vi "AlliGator 2-Exp + IRF Convolution Fit v2.vi"(0 "Decay":cluster{"t Array":dbl[], "Data Array":dbl[]}, 5 "IRF":cluster{"t Array":dbl[], "IRF Array":dbl[]}, 9 "Fit Options":T9={"Show Fit Residuals"=TRUE, "Fit Model"=enum."1-Exponential", "Residual Type"=enum."Standard", "Max Decay Percentile"=0.0, "Min Decay Percentile"=0.0, "Show Full Decay"=TRUE, "Weights"=enum."Unweighted", "Fitting Method"=enum."Least Square", "Compute Parameter Uncertainties"=TRUE, "Periodic Boundaries"=TRUE, "Model Calculation"=enum."Simulation", "Period"=1.2500000000000001e-08, "Termination Criteria"={"Max Iterations"=1000, "Max Function Calls"=0, "Max Time"=1000.0, "Function Tolerance"=1e-06, "Parameter Tolerance"=1e-06, "Gradient Tolerance"=0.0, "Min Lambda"=1e-06, "Max Lambda"=1e-06, "Initial Tick Count"=0}, "Offset Resolution"=1.2500000000000001e-08, "Use Local IRF"=TRUE, "Fitting Algorithm"=enum."Levenberg-Marquardt"} {"Offset Resolution" min=0.0; "Period" min=0.0; "Min Decay Percentile" min=0.0 max=1.0; "Max Decay Percentile" min=0.0 max=100.0}, 11 "error in (no error)":errorcluster, 12 "parameter bounds":T8) -> (4 "Fitted Decay":cluster{"t Array":dbl[], "Fitted Array":dbl[]}, 6 "Residuals":cluster{"t Array":dbl[], "Residual Array":dbl[]}, 8 "Fit Output":T2={"best nonlinear fit"=[], "best fit parameters"=[], "R^2"=0.0, "RMSE"=0.0, "error out"={"status"=FALSE, "code"=0, "source"=""}, "Fitting Method"=enum."Least Square", "number of function calls"=0, "number of iterations"=0, "covariance"=[], "Chi 2"=0.0, "DOF"=0, "Fit Convergence Criterion"=enum."Continue", "Fitting Algorithm"=enum."Levenberg-Marquardt", "Weighted Fit"=FALSE, "Gradient"=0.0, "|Delta Chi 2|"=0.0, "|Delta Chi 2|/Chi 2"=0.0, "Max |Delta a| /|a|"=0.0, "Lambda"=-1.0, "RSS"=0.0, "AIC"=0.0, "BIC"=0.0, "Max number of function calls"=0, "Max number of iterations"=0, "IRF"={"X Array"=[], "Y Array"=[]}, "IRF Normalization Factor"=0.0, "Decay Normalization Factor"=0.0}, 10 "Delta Best Fit Parameters":dbl[](array[numeric]), 13 "Guess Parameters Options":T1=enum."User-provided (normalized)", 14 "Guess Parameters":dbl[](array[numeric]), 15 "error out":errorcluster)   [LabVIEW 2021, in "AlliGator Decay Analysis.lvlib" / "AlliGator Decay Fit.lvlib"]
doc: "Legacy code for 2-Exp decay fit."
uses:
  AlliGator Decay Fit.lvlib
  Fits/IRF(X)PSED/Decay Fit Options v2.ctl
  Fits/Decay Convolution/Decay Model.ctl
  Fits/Residual Type.ctl
  Fits/IRF(X)PSED/Fit Weights Type.ctl
  Fits/Non-linear Fitting Method v2.ctl
  Fits/Fit Calculation Method.ctl
  Fits/Non-linear Fitting Algorithm.ctl
  Fits/Non-linear Fit Output v3.ctl
  Fits/Nonlinear Fit Method.ctl
  <vilib>/Analysis/Matrix/Datatypes/RealMatrix.ctl
  Fits/Convergence Criteria.ctl
  Graphs/XY Graph/XY Plot Data.ctl
  AlliGator Guess Parameters Options.ctl
  AlliGator Settings List.ctl
  Fits/Decay Convolution/Fit Control Data.ctl
  AlliGator Variables List.ctl
  Fits/Decay Convolution/LM model function and gradient (2-Exp + IRF) v2.vi
  Phasor/Phasor Abort Parallel Computation.vi
  Fits/Decay Convolution/LM model function and gradient (2-Exp, Convolved, Periodic) v3.vi
  <vilib>/Utility/error.llb/Error Cluster From Error Code.vi
  Fits/Abort Fit Global.vi
  <vilib>/ErrorRing/Error Ring.xnode
  Time/Time.lvlib
  Fits/Fits.lvlib
  AlliGator Settings.lvlib
  Phasor/Phasor.lvlib
  AlliGator Globals, Variables & Constants.lvlib
  Error/Error.lvlib
  Graphs/XY Graph/XY Graph Add-Ons.lvlib
  <vilib>/Analysis/Matrix/NI_Matrix.lvlib
panel:
  out "CPU (s)":dbl
  out "XY Graph":T15(graph)
  # "Offset\nBaseline\nA1\ntau1\nA2\ntau2"
  # "Offset\nBaseline\nA1\ntau 1\nA2\ntau 2"
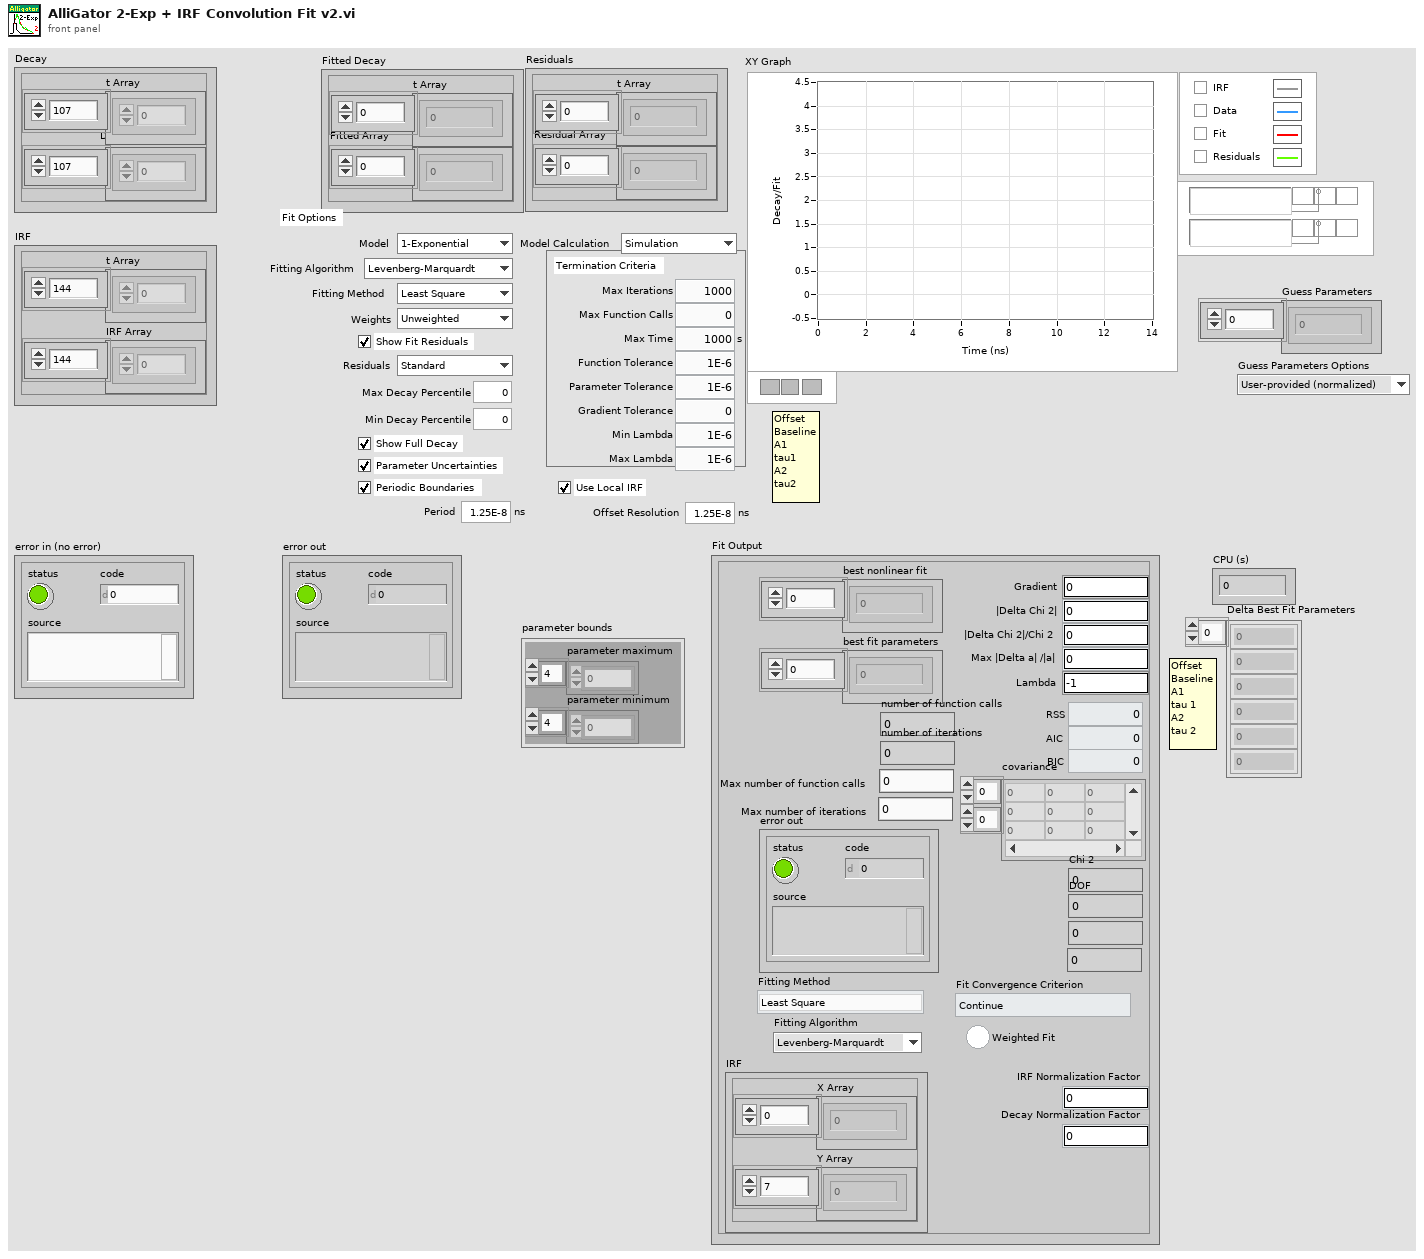
[diagram p1: front panel]
types:
  T1 = typedef "AlliGator Decay Analysis.lvlib/AlliGator Decay Fit.lvlib/AlliGator Guess Parameters Options.ctl" = enum16{"Numerically estimated", "User-provided", "User-provided (normalized)", "Last valid fitted parameters"}
  T2 = typedef "Fits.lvlib/Non-linear Fit Output v3.ctl" = cluster{"best nonlinear fit":dbl[], "best fit parameters":dbl[], "R^2":dbl, "RMSE":dbl, "error out":errorcluster, "Fitting Method":T3, "number of function calls":i32, "number of iterations":i32, "covariance":T4, "Chi 2":dbl, "DOF":i32, "Fit Convergence Criterion":T5, "Fitting Algorithm":T6, "Weighted Fit":bool, "Gradient":dbl, "|Delta Chi 2|":dbl, "|Delta Chi 2|/Chi 2":dbl, "Max |Delta a| /|a|":dbl, "Lambda":dbl, "RSS":dbl, "AIC":dbl, "BIC":dbl, "Max number of function calls":i32, "Max number of iterations":i32, "IRF":T7, "IRF Normalization Factor":dbl, "Decay Normalization Factor":dbl}
  T3 = typedef "Fits.lvlib/Nonlinear Fit Method.ctl" = enum16{"Least Square", "Least Absolute Residual", "Bisquare", "MLE"}
  T4 = typedef "NI_Matrix.lvlib/RealMatrix.ctl" = dbl[][]
  T5 = typedef "Fits.lvlib/Convergence Criteria.ctl" = enum16{"Continue", "Tolerances Exceeded", "Max Time Exceeded", "Max Iterations Exceeded", "Max Function Evaluations Exceeded", "Scale Range Exceeded"}
  T6 = typedef "Fits.lvlib/Non-linear Fitting Algorithm.ctl" = enum16{"Levenberg-Marquardt", "Trust-Region Dogleg"}
  T7 = typedef "XY Graph Add-Ons.lvlib/XY Plot Data.ctl" = cluster{"X Array":dbl[], "Y Array":dbl[]}
  T8 = cluster{"parameter minimum":dbl[], "parameter maximum":dbl[]}
  T9 = typedef "Fits.lvlib/Decay Fit Options v2.ctl" = cluster{"Show Fit Residuals":bool, "Fit Model":T10, "Residual Type":T11, "Max Decay Percentile":dbl, "Min Decay Percentile":dbl, "Show Full Decay":bool, "Weights":T12, "Fitting Method":T13, "Compute Parameter Uncertainties":bool, "Periodic Boundaries":bool, "Model Calculation":T14, "Period":dbl[unit], "Termination Criteria":cluster{"Max Iterations":i32, "Max Function Calls":i32, "Max Time":dbl[unit], "Function Tolerance":dbl, "Parameter Tolerance":dbl, "Gradient Tolerance":dbl, "Min Lambda":dbl, "Max Lambda":dbl, "Initial Tick Count":u32}, "Offset Resolution":dbl[unit], "Use Local IRF":bool, "Fitting Algorithm":T6}
  T10 = typedef "Fits.lvlib/Decay Model.ctl" = enum16{"1-Exponential", "2-Exponentials"}
  T11 = typedef "Fits.lvlib/Residual Type.ctl" = enum16{"Standard", "Normalized", "Reduced"}
  T12 = typedef "Fits.lvlib/Fit Weights Type.ctl" = enum16{"Unweighted", "1/Variance", "Best of All"}
  T13 = typedef "Fits.lvlib/Non-linear Fitting Method v2.ctl" = enum16{"Least Square", "Least Absolute Residual", "Bisquare", "MLE", "-", "Best of All"}
  T14 = typedef "Fits.lvlib/Fit Calculation Method.ctl" = enum16{"Simulation", "Convolution", "Integration"}
  T15 = cluster{"t Array":dbl[], "best nonlinear fit":dbl[]}[]
  T16 = typedef "AlliGator Settings.lvlib/AlliGator Settings List.ctl" = enum16{"GUI:Visible Settings Tab", "GUI:Last Run Version", "Source Image:Use Image Histogram for Contrast", "Source Image:Low Count Pixels Rejection Options", "Source Image:High Count Pixels Rejection Options", "Source Image:Use Image Brightness", "Source Image:Blend Overlay with Image Background", "Source Image:Use Fixed ROI Diameter", "Source Image:ROI Diameter", "Source Image:ROI Center Color", "Source Image:Peak Threshold", "Source Image:Intensity Threshold", "Source Image:Image Binning Options", "Source Image:Image Smoothing Options", "Source Image:Image Histogram Active", "Source Image:Invert Binary Mask", "Source Image:Hot Pixel Removal", "Source Image:Overlay Analyzed ROI Center", "Source Image:Auto-Adjust Contrast", "Source Image:Histogram Lower Percentile", "Source Image:Histogram Upper Percentile", "Source Image:Save Source Image", "Source Image:Scale Bar Options", "Source Image:Image Resolution (Pixel Size)", "Source Image:Flatfield Correction", "Source Image:Show Dead Left Columns Correction", "Source Image:Dead Left Columns Correction", "Source Image:Image Pre-Processing Operations Order", "Source Image:Overlay ROI Median", "Source Image:Median Overlay Color", "Data Information:Gate Width", "Data Information:Nanotime Gate Separation", "Data Information:Macrotime Gate Separation", "Data Information:Gate Step", "Data Information:# Gates", "Data Information:Gate Image Exposure", "Data Information:Gate Image Integration", "Data Information:Gates to Skip", "Data Information:Gates to Keep", "Data Information:Define Gates to", "Data Information:Channel Name", "Data Information:Available Channel Names", "Data Information:Channel Arithmetic", "Data Information:Background File Subtraction", "Data Information:Background File", "Data Information:Background Scaling Factor", "Data Information:Background Pile-up Correction", "Data Information:Background Pixel Well Capacity", "Data Information:Laser Period", "Data Information:SYNC Period", "Data Information:Pile-up Correction", "Data Information:Pixel Well Capacity", "Data Information:Dataset Scaling Factor", "Fluorescence Decay_Decay Pre-Processing:Reverse Gates", "Fluorescence Decay_Decay Pre-Processing:Verbose Decay Pre-Processing", "Fluorescence Decay_Decay Pre-Processing:Use Decay Pre-Processing", "Fluorescence Decay_Decay Pre-Processing:Background Subtraction", "Fluorescence Decay_Decay Pre-Processing:Background Definition Range", "Fluorescence Decay_Decay Pre-Processing:Baseline Subtraction Method", "Fluorescence Decay_Decay Pre-Processing:Decay Pre-Processing Operations Order", "Fluorescence Decay_Decay Pre-Processing:Smoothing Parameter", "Fluorescence Decay_Decay Pre-Processing:Shift Decay", "Fluorescence Decay_Decay Pre-Processing:Decay Shift Parameters", "Fluorescence Decay_Decay Pre-Processing:Fold Decay", "Fluorescence Decay_Decay Pre-Processing:# Folds", "Fluorescence Decay_Decay Pre-Processing:1-Normalize Decay", "Fluorescence Decay_Decay Pre-Processing:[0-1]-Normalize Decay", "Fluorescence Decay_Decay Pre-Processing:Smoothen Decay", "Fluorescence Decay_Decay Pre-Processing:Extrapolate Decay", "Fluorescence Decay_Decay Pre-Processing:Use Periodicity", "Fluorescence Decay_Decay Pre-Processing:Use Cursors", "Fluorescence Decay_Decay Pre-Processing:Tail Fraction", "Fluorescence Decay_Decay Pre-Processing:Head Fraction", "Fluorescence Decay_Decay Pre-Processing:Additional Points", "Fluorescence Decay_Decay Pre-Processing:Straighten Decay", "Fluorescence Decay_Decay Pre-Processing:Constant Background", "Fluorescence Decay_Decay Pre-Processing:Pixel-Normalize Decay", "Fluorescence Decay_Advanced Analysis:Extract IRF instead of Decay", "Fluorescence Decay_Advanced Analysis:IRF Extraction Options", "Fluorescence Decay_Advanced Analysis:IRF Optimization Options", "Fluorescence Decay_Advanced Analysis:Square Pulse Options", "Fluorescence Decay_Advanced Analysis:IRF Order", "Fluorescence Decay_Advanced Analysis:IRF Time Constants", "Fluorescence Decay_Advanced Analysis:Wavelet Analysis Options", "Fluorescence Decay_Advanced Analysis:Average Lifetime Options", "Fluorescence Decay_Fit Options:Fit Options", "Fluorescence Decay_Fit Options:Use Legacy Fitting Approach", "Fluorescence Decay_Fit Options:Use Data Information Laser Period", "Fluorescence Decay_Fit Parameters:Displayed Fit Parameters", "Fluorescence Decay_Fit Parameters:Fit Parameter Constraints", "Fluorescence Decay_Fit Parameters:Export Tabulated Results", "Fluorescence Decay_Fit Parameters:MLE Baseline Offset Type", "Fluorescence Decay_Fit Parameters:MLE Baseline Offset", "Fluorescence Decay_Fit Parameters:Guess Parameter Names", "Fluorescence Decay_Fit Parameters:Guess Parameter Values", "Fluorescence Decay_Fit Parameters:Guess Parameters Options", "Fluorescence Decay_Styles:Show Last Decay Only", "Fluorescence Decay_Styles:Decay Graph Color Array", "Fluorescence Decay:Decay Graph Active", "Fluorescence Decay Statistics:Min Peak Value", "Fluorescence Decay Statistics:Reject Low Decay Peak Pixels", "Fluorescence Decay Statistics:Reject High Decay Peak Pixels", "Fluorescence Decay Statistics:Max Peak Value", "Time Traces:Use File Timestamp", "Time Traces:Time Step", "Time Traces:Use Intensity Correction File", "Time Traces:Intensity Correction File", "Phasor Plot:Phasor Plot Smoothing Options", "Phasor Plot:Phasor Plot Size", "Phasor Plot:Phasor Plot Graphics Options", "Phasor Plot:Cumulative Phasor Plot", "Phasor Plot:Use Phasor Brightness", "Phasor Plot:Blend Overlay with Phasor Background", "Phasor Plot:Save Phasor Plot", "Phasor Plot:Show References", "Phasor Plot:Phasor Ratio Decay Range", "Phasor Plot:Exponential Fading", "Phasor Plot:Phasor Ratio Reference Colors", "Phasor Plot:Reference Radius", "Phasor Plot:Show Color Map Vertices", "Phasor Plot:Phasor Plot Active", "Phasor Plot:Phasor Ratio Color Map Type", "Phasor Plot:Phasor Ratio Color Map", "Phasor Plot:Phasor Ratio Display Range", "Phasor Plot:Selected Image ROI(s)", "Phasor Plot:All Image ROIs", "Phasor Plot:Selected Phasor Plot ROI(s)", "Phasor Plot:All Phasor Plot ROIs", "Phasor Plot:Phasor Ratio Color-Coded Quantity", "Phasor Plot:Store Phasor Harmonics", "Phasor Plot:Draw Reference Segment", "Phasor Plot:User-Defined Quantity", "Phasor Graph:Phasor Frequency", "Phasor Graph:Phasor Ratio Type", "Phasor Graph:Pixel-level Phasor Computation", "Phasor Graph:Save Phasor Graph", "Phasor Graph:Phasor Graph Active", "Phasor Graph:Phasor SDV Options", "Phasor Calibration:Use Backup Calibration if needed", "Phasor Graph:Define Shortest Lifetime as", "Phasor Calibration:Backup Calibration Type", "Phasor Calibration:Calibration Type", "Phasor Calibration:Calibration Lifetime", "Phasor Calibration:Calibration Map Algorithm", "Single-Exponential Phasor Locus (SEPL):Gate Parameters", "Single-Exponential Phasor Locus (SEPL):User-defined Gate", "Single-Exponential Phasor Locus (SEPL):User-defined IRF", "Single-Exponential Phasor Locus (SEPL):Phasor Parameters", "Single-Exponential Phasor Locus (SEPL):Decay & IRF Parameters", "Single-Exponential Phasor Locus (SEPL):Display Parameters", "Lifetime Analysis:Decay Analysis Parameters", "Lifetime Analysis:Lifetime Map Active", "Plugins:Python Settings", "Miscellaneous:Verbose Mode", "Miscellaneous:Beep after Script", "Miscellaneous:Saved Image File Format", "Miscellaneous:Exported Gate Image Settings", "Miscellaneous:Include Loading in Timing", "Miscellaneous:Verbose Settings Mode", "Miscellaneous:Histogram Options", "Miscellaneous:Beep on Error", "Miscellaneous:# Logical Processors Used", "Miscellaneous:ROI Description Max Characters", "Miscellaneous:Verbose Error Mode", "Miscellaneous:Transparent Mask Color"}
  T17 = typedef "Fits.lvlib/Fit Control Data.ctl" = cluster{"IRF":T7, "Laser Period":dbl, "SYNC Period":dbl}
  T18 = typedef "Fits.lvlib/Decay Fit Parameters In List.ctl" = enum16{"Offset", "Baseline", "A_1", "tau_1", "A_2", "tau_2"}
  T19 = typedef "Fits.lvlib/Fit Results (statistics).ctl" = cluster{"Chi2/DOF":dbl, "R2":dbl, "RMSE":dbl, "Fitting Method":T13, "Fitting Algorithm":T6}
  T20 = typedef "AlliGator Globals, Variables & Constants.lvlib/AlliGator Variables List.ctl" = enum16{"---- GUI ----", "GUI:Initialization Status", "GUI:State Indicators Refnum", "GUI:Original AlliGator Menu Items", "GUI:Current Action Loop State", "GUI:Script in progress", "GUI:Playback", "GUI:Loop Playback", "GUI:Search ROI Used", "GUI:Search ROI", "Decay Graph Max Legend Size", "Intensity Graph Max Legend Size", "Decay Statistics Graph Max Legend Size", "Phasor Graph Max Legend Size", "Phasor Ratio Graph Max Legend Size", "Lifetime Graph Max Legend Size", "---- Files ----", "Files:Export Dataset Frames as Individual Files", "Files:Show Batch Export Help Balloons", "Files:Frames in Dataset", "Files:ptu File Frame Start Indices", "Files:Current Frame in Dataset", "Files:Current Frame Timestamp", "Files:Dataset Loaded", "Files:Dataset Metadata", "Files:Dataset Channel", "Files:Dataset Data Description", "Files:Background Dataset Metadata", "Files:Background Dataset Channel", "Files:Background Dataset Data Description", "Files:Background File Subtraction", "Files:Background File Path", "Files:Background File Pile-up Correction", "Files:Background File Pixel Well Capacity", "Files:Background File Scaling Factor", "Files:Current Dataset Load Settings", "Files:Dataset Path", "Files:ICCD-specific Information", "Files:Macrotime Gate Separation", "------ Python Plugins ------", "Python Plugins:Information", "Python Plugins:Python Session", "Python Plugins:Valid Python Session?", "---- Source Image ----", "Source Image:ROIs", "Source Image:Current ROI", "Source Image:ROI Event Refnum", "X_Source Image Display Range", "X_Source Image Palette Information", "X_Type of Displayed Image", "X_Time Gate Slider", "Source Image:Palette List", "Source Image:Scale", "Source Image:ROI Overlay Color", "Source Image:Overlay to Erase", "Source Image:Is Displayed Image Accumulated", "Source Image:White Light Image Modified", "Source Image:Mask Image Modified", "---- Image Profile Window ----", "Image Profile:Window Event Refnum", "Image Profile:IntensityType", "Image Profile:Intensity Average Type", "Image Profile:Intensity-weighted SDV", "Image Profile:Box Profile Type", "Image Profile:Window Open", "Image Profile:Plotted Fit Parameter", "------ Phasor Graph -------", "Phasor Graph:Show Line", "---- Phasor Plot ---", "Phasor Plot:Parameters Changed", "Phasor Plot:FLI Dataset Modified since last Calculation", "Phasor Harmonics Data", "Selected Phasor Harmonics", "Phasor Harmonic Manager Event Refnum", "Phasor Plot:ROIs", "Phasor Plot:Current ROI", "Phasor Plot:ROI Event Refnum", "Phasor Plot:Image Reference Points", "Phasor Plot:Computed", "Phasor Plot:Palette Information", "Phasor Plot:Palette List", "Phasor Plot:Phasor Ratio Palette Information", "Phasor Plot:Phasor Ratio Palette List", "Phasor Plot:Image Scale", "Phasor Plot:Image Overlay to Erase", "Phasor Plot:Image Elements to Update", "Phasor Plot:Current Calculation Parameters", "Phasor Plot:Current Calibration Options", "Phasor Plot:Reset Cumulated Phasor Plot", "Phasor Plot:Reference 1", "Phasor Plot:Lifetime Reference 1", "Phasor Plot:Reference 1 Frequency", "Phasor Plot:Reference 2", "Phasor Plot:Lifetime Reference 2", "Phasor Plot:Reference 2 Frequency", "---- Decay Analysis ----", "Number of Selected Decays to Fit", "LS Fit Results", "LAR Fit Results", "BS Fit Results", "Last Decay Max - Min", "Best Fit Parameters", "Best Fit Parameter Names", "Actual Size X", "Actual Size Y", "Binning X", "Binning Y", "Actual # Gates", "Dataset Number", "Gates to...", "Gates Skipped", "Gates to keep", "Gate Step", "Gate Separation", "Reversed Gates", "Pile-up Correction", "Pixel Well Capacity", "Background Subtracted", "Background Subtraction Method", "Background Definition Range", "Background File (deprecated)", "Number of Dataset Accumulated", "Array of Accumulated Dataset Paths", "Do Averaged Datasets", "Destination File Path", "Process Plot Target", "Use 1/D as Phasor Frequency", "---- Decay Fit Parameter Map -----", "Decay Fit Parameter Map:Palette Information", "Decay Fit Parameter Map:Palette List", "------- Local Decay Window ---------", "Local Decay Graph Window:Event Refnum", "Local Decay Graph Window:Use normalized IRF for convolution", "----- Miscellaneous ----", "Misc:Skippable Dialog Windows Status"}
  T21 = cluster{"t Array":dbl[], "best nonlinear fit":dbl[]}
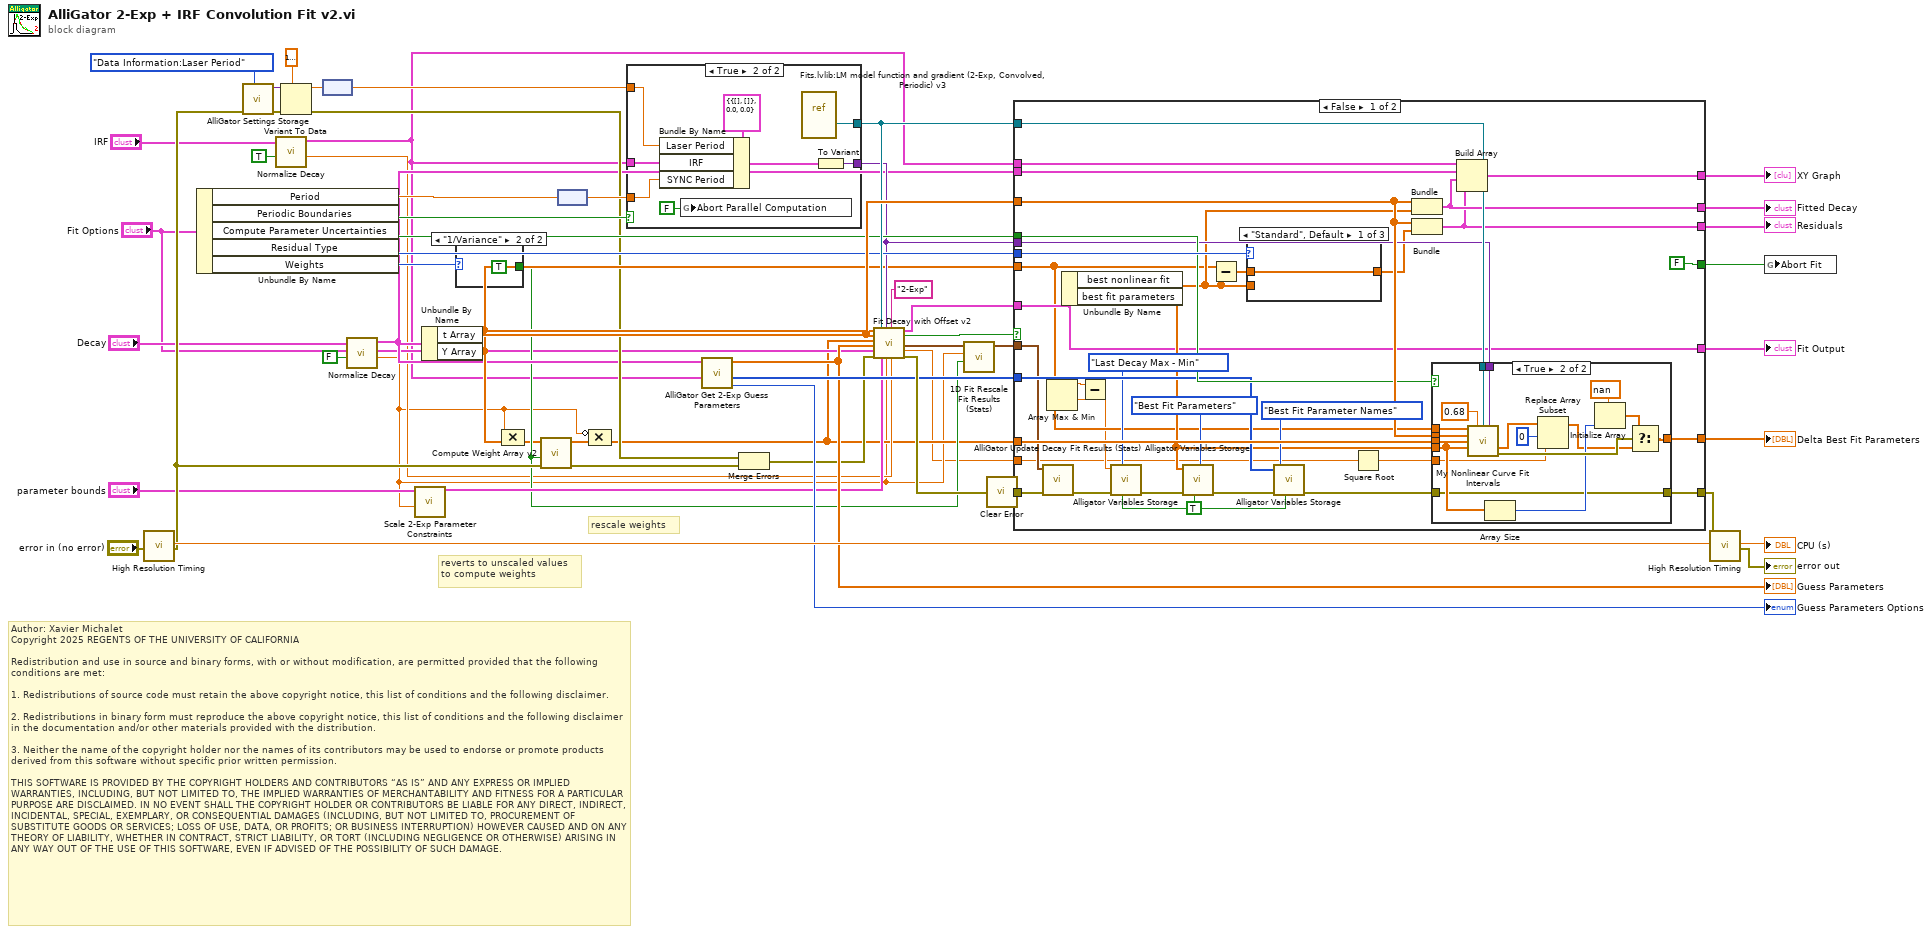
[diagram p0: block diagram]
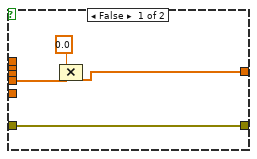
[diagram p3: hidden frame]
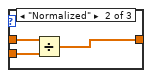
[diagram p4: hidden frame]
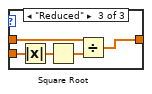
[diagram p5: hidden frame]
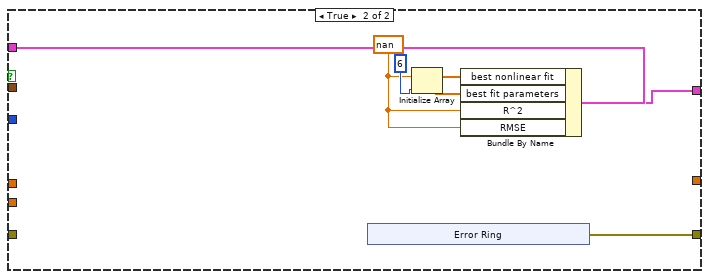
[diagram p6: hidden frame]
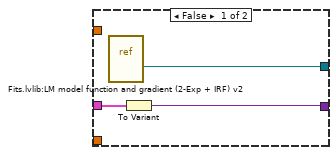
[diagram p7: hidden frame]
diagram:
  # "Author: Xavier Michalet\nCopyright 2025 REGENTS OF THE UNIVERSITY OF CALIFORNIA\n\nRedistribution and use in source and binary forms, with or without modification, are permitted provided that the following conditions are met:\n\n1. Redistributions of source code must retain the above copyright notice, this list of conditions and the following disclaimer.\n\n2. Redistributions in binary form must reproduce the above copyright notice, this list of conditions and the following disclaimer in the documentation and/or other materials provided with the distribution.\n\n3. Neither the name of the copyright holder nor the names of its contributors may be used to endorse or promote products derived from this software without specific prior written permission.\n\nTHIS SOFTWARE IS PROVIDED BY THE COPYRIGHT HOLDERS AND CONTRIBUTORS “AS IS” AND ANY EXPRESS OR IMPLIED WARRANTIES, INCLUDING, BUT NOT LIMITED TO, THE IMPLIED WARRANTIES OF MERCHANTABILITY AND FITNESS FOR A PARTICULAR PURPOSE ARE DISCLAIMED. IN NO EVENT SHALL THE COPYRIGHT HOLDER OR CONTRIBUTORS BE LIABLE FOR ANY DIRECT, INDIRECT, INCIDENTAL, SPECIAL, EXEMPLARY, OR CONSEQUENTIAL DAMAGES (INCLUDING, BUT NOT LIMITED TO, PROCUREMENT OF SUBSTITUTE GOODS OR SERVICES; LOSS OF USE, DATA, OR PROFITS; OR BUSINESS INTERRUPTION) HOWEVER CAUSED AND ON ANY THEORY OF LIABILITY, WHETHER IN CONTRACT, STRICT LIABILITY, OR TORT (INCLUDING NEGLIGENCE OR OTHERWISE) ARISING IN ANY WAY OUT OF THE USE OF THIS SOFTWARE, EVEN IF ADVISED OF THE POSSIBILITY OF SUCH DAMAGE."
  # "rescale weights"
  # "reverts to unscaled values to compute weights"
  n1 = call "High Resolution Timing.vi"("Error In"="error in (no error)") -> ("elapsed (relative) seconds"=w56:dbl, "Error Out"=w28:errorcluster)  [unwired: 16 in, 1 out]
  n2 = Unbundle By Name("Fit Options") -> ("Period"=w34:dbl[unit], "Periodic Boundaries"=w44:bool, "Compute Parameter Uncertainties"=w45:bool, "Residual Type"=w52:T11, "Weights"=w20:T12)
  n3 = call "AlliGator Settings Storage.vi"("AlliGator Settings List"=AlliGator_Settings_List."Data Information:Laser Period", "Error In"=w28) -> ("Error Out"=w30:errorcluster, "Variant Data out"=w42:variant)  [unwired: 8 in]
  n4 = call "Normalize Decay.vi"("IRF (F)"=TRUE, "Decay"="IRF") -> ("Normalization Factor"=w5:dbl, "Normalized Decay"=w7:cluster{"t Array":dbl[], "Y Array":dbl[]})  [unwired: 7 in, 1 out]
  n5 = Variant To Data(error in=w30, type=dbl[unit] 1e-09 ("New"), Variant=w42) -> (data=w40:dbl[unit], error out=w26:errorcluster)
  n6 = node(w40) -> (w38:dbl)
  n7 = call "Normalize Decay.vi"("IRF (F)"=FALSE, "Decay"="Decay") -> ("Normalization Factor"=w2:dbl, "Normalized Decay"=w17:cluster{"t Array":dbl[], "Y Array":dbl[]})  [unwired: 7 in, 1 out]
  n8 = call "Scale 2-Exp Parameter Constraints.vi"("Normalization Factor"=w2, "parameter bounds in"="parameter bounds") -> ("parameter bounds out"=w13:T8)  [unwired: 9 in]
  n9 = Unbundle By Name(w17) -> ("t Array"=w54:dbl[], "Y Array"=w31:dbl[])
  n10 = case shown="\"1/Variance\"" w20 {
    tunnel: [_ TRUE ("Weighted Fit")] -> w11
    frame "Unweighted", Default {
    }
    frame "1/Variance" {
    }
  }
  n11 = Compound Arithmetic op=MULTIPLY(w2, w31) -> (w4:dbl[])
  n12 = call "Compute Weight Array v2.vi"("Error In"=w28, "Weighted Fit"=w11, "Data Array"=w4) -> ("Error Out"=w27:errorcluster, "Weight Array"=w24:dbl[])  [unwired: 7 in]
  n13 = node(w34) -> (w33:dbl)
  n14 = Compound Arithmetic op=MULTIPLY(invert w2, w24) -> (w3:dbl[])
  n15 = case shown="True" w44 {
    tunnel: [w61 w69] -> w53
    tunnel: w7 -> [w60 w67]
    tunnel: [w59 w65] -> w39
    tunnel: w38 -> [_ w63]
    tunnel: w33 -> [_ w62]
    frame False {
      n16 = vi-ref "Fits.lvlib:LM model function and gradient (2-Exp + IRF) v2.vi"() -> (w61:refnum<vi>)
      n17 = To Variant(anything=w60) -> (Variant=w59:variant)
    }
    frame True {
      n18 = Bundle By Name(cluster=T17 {"IRF"={"X Array"=[], "Y Array"=[]}, "Laser Period"=0.0, "SYNC Period"=0.0}, "Laser Period"=w63, "IRF"=w67, "SYNC Period"=w62) -> (w66:T17)
      n19 = global write "Phasor Abort Parallel Computation.vi" "Abort Parallel Computation"(FALSE ("Abort Parallel Computation")) -> ()
      n20 = vi-ref "Fits.lvlib:LM model function and gradient (2-Exp, Convolved, Periodic) v3.vi"() -> (w69:refnum<vi>)
      n21 = To Variant(anything=w66) -> (Variant=w65:variant)
    }
  }
  n22 = call "AlliGator Get 2-Exp Guess Parameters.vi"("IRF"=w7, "Decay"=w17) -> ("Guess Parameters Type"=→"Guess Parameters Options":T1, "Guess Parameters Names"=w37:T18[], "Guess Parameters"=w35:dbl[])  [unwired: 7 in]
  "Guess Parameters" <- w35
  n23 = Merge Errors(w26, w27) -> (w25:errorcluster)
  n24 = call "Fit Decay with Offset v2.vi"("Y Array"=w31, "X Array"=w54, "Weights"=w3, "Initial Parameters"=w35, "Decay Fit Options"="Fit Options", "error in (no error)"=w25, "f(x,a)"=w53, "parameter bounds"=w13, "Data"=w39, "Decay Normalization Factor"=w2, "Model Name"="2-Exp", "IRF Normalization Factor"=w5) -> ("Fit Output"=w16:T2, "Fit Aborted?"=w32:bool, "Fit Results (Stats)"=w12:T19[], "C_00"=w1:dbl, "error out"=w46:errorcluster)  [unwired: 3 in]
  n25 = call "1D Fit Rescale Fit Results (Stats).vi"("Weighted"=w11, "Normalization Factor"=w2, "Fit Results (Stats) in"=w12) -> ("Fit Results (Stats) out"=w10:T19[])  [unwired: 8 in]
  n26 = call "Clear Error.vi"("Error In"=w46) -> ("no Error Out"=w22:errorcluster)  [unwired: 8 in]
  n27 = case shown="False" w32 {
    tunnel: w31 -> [w77 _]
    tunnel: w54 -> [w105 _]
    tunnel: w53 -> [w104 _]
    tunnel: w52 -> [w103 _]
    tunnel: [w102 _] -> w51
    tunnel: [w101 _] -> w50
    tunnel: [w100 _] -> w49
    tunnel: [w99 _] -> w48
    tunnel: [w98 w141] -> w47
    tunnel: w22 -> [w97 _]
    tunnel: w3 -> [w96 _]
    tunnel: w16 -> [w82 w137]
    tunnel: w45 -> [w95 _]
    tunnel: w17 -> [w94 _]
    tunnel: w7 -> [w93 _]
    tunnel: w39 -> [w92 _]
    tunnel: w37 -> [w91 _]
    tunnel: [w82 w136] -> w23
    tunnel: w10 -> [w73 _]
    tunnel: [FALSE ("Abort Fit") _] -> w6
    tunnel: w1 -> [w71 _]
    frame False {
      w79 = TRUE ("Get(F)/Set")
      n28 = call "AlliGator Update Decay Fit Results (Stats).vi"("error in (no error)"=w97, "Fit Results"=w73) -> ("error out"=w81:errorcluster)  [unwired: 9 in]
      n29 = Array Max & Min(array=w77) -> (max value=w76:dbl, min value=w75:dbl)  [unwired: 2 out]
      n30 = Unbundle By Name(w82) -> ("best nonlinear fit"=w88:dbl[], "best fit parameters"=w83:dbl[])
      n31 = Subtract(x=w76, y=w75) -> (x-y=w74:dbl)
      n32 = call "Alligator Variables Storage.vi"("Get(F)/Set"=w79, "AlliGator Variable"=AlliGator_Variables_List."Last Decay Max - Min" ("Alligator Variable"), "Error In"=w81, "Data in"=w74) -> ("Error Out"=w80:errorcluster)  [unwired: 5 in, 2 out]
      n33 = call "Alligator Variables Storage.vi"("Get(F)/Set"=w79, "AlliGator Variable"=AlliGator_Variables_List."Best Fit Parameters" ("Alligator Variable"), "Error In"=w80, "Data in"=w83) -> ("Error Out"=w87:errorcluster)  [unwired: 5 in, 2 out]
      n34 = Subtract(x=w77, y=w88) -> (x-y=w90:dbl[])
      n35 = case shown="\"Standard\", Default" w103 {
        tunnel: w90 -> [w127 w130 w135]
        tunnel: [w127 w128 w133] -> w89
        tunnel: w88 -> [_ w129 w134]
        frame "Standard", Default {
        }
        frame "Normalized" {
          n36 = Divide(x=w130, y=w129) -> (x/y=w128:dbl[])
        }
        frame "Reduced" {
          n37 = Absolute Value(x=w134) -> (abs(x)=w132:dbl[])
          n38 = Square Root(x=w132) -> (sqrt(x)=w131:dbl[])
          n39 = Divide(x=w135, y=w131) -> (x/y=w133:dbl[])
        }
      }
      n40 = call "Alligator Variables Storage.vi"("Get(F)/Set"=w79, "AlliGator Variable"=AlliGator_Variables_List."Best Fit Parameter Names" ("Alligator Variable"), "Error In"=w87, "Data in"=w91) -> ("Error Out"=w84:errorcluster)  [unwired: 5 in, 2 out]
      n41 = Square Root(x=w71) -> (sqrt(x)=w70:dbl)
      n42 = Bundle("t Array"=w105, "best nonlinear fit"=w88) -> (w101:T21)  [unwired: 1 in]
      n43 = Bundle("t Array"=w105, w89) -> (w100:cluster{"t Array":dbl[], dbl[]})  [unwired: 1 in]
      n44 = case shown="True" w95 {
        tunnel: [w109 w113] -> w98
        tunnel: [w108 w118] -> w99
        tunnel: w105 -> [_ w125]
        tunnel: w104 -> [_ w124]
        tunnel: w96 -> [_ w123]
        tunnel: w92 -> [_ w122]
        tunnel: w83 -> [w106 w115]
        tunnel: w77 -> [_ w121]
        tunnel: w84 -> [w109 w113]
        tunnel: w70 -> [_ w110]
        frame False {
          n45 = Compound Arithmetic op=MULTIPLY(0.0, w106) -> (w108:dbl[])
        }
        frame True {
          n46 = call "My Nonlinear Curve Fit Intervals.vi"("Y"=w121, "confidence level"=0.68, "f(x,a)"=w124, "data"=w122, "X"=w125, "Weight"=w123, "best fit parameters"=w115) -> ("delta best fit parameters"=w120:dbl[], "error out"=w119:errorcluster)  [unwired: 7 in]
          n47 = Array Size(array=w115) -> (size(s)=w114:i32)
          n48 = Replace Array Subset(array=w120, new element=w110, index=0) -> (w112:dbl[])
          n49 = Initialize Array(nan ("element"), w114) -> (w116:dbl[])
          n50 = Select(t=w116, s=w119, f=w112) -> (s? t:f=w118:dbl[])
        }
      }
      n51 = Build Array(w93, w94, w101, w100) -> (w102:T15)
    }
    frame True {
      w139 = nan ("element")
      n52 = xnode "Error Ring"() -> ("error out"=w141:errorcluster)
      n53 = Initialize Array(w139, 6 ("dimension size")) -> (w138:dbl[])
      n54 = Bundle By Name(cluster=w137, "best nonlinear fit"=w138, "best fit parameters"=w138, "R^2"=w139, "RMSE"=w139) -> (w136:T2)
    }
  }
  "Fitted Decay" <- w50
  "XY Graph" <- w51
  "Delta Best Fit Parameters" <- w48
  "Residuals" <- w49
  "Fit Output" <- w23
  n55 = call "High Resolution Timing.vi"("relative seconds (NaN)"=w56, "Error In"=w47) -> ("elapsed (relative) seconds"=→"CPU (s)":dbl, "Error Out"=→"error out":errorcluster)  [unwired: 15 in, 1 out]
  n56 = global write "Abort Fit Global.vi" "Abort Fit"(w6) -> ()
